vi "Enque Epics Message Bool Array.vi"(7 "Message name":string, 8 "error in (no error)":errorcluster, 9 "Numeric":u32, 10 "Epics variable":bool[](array[boolean]), 11 "Queue in":refnum<queue>) -> (0 "error out":errorcluster)   [LabVIEW 2014]
uses:
  Message Queue/Message Cluster.ctl
  Message Queue/Message Queue.lvlib
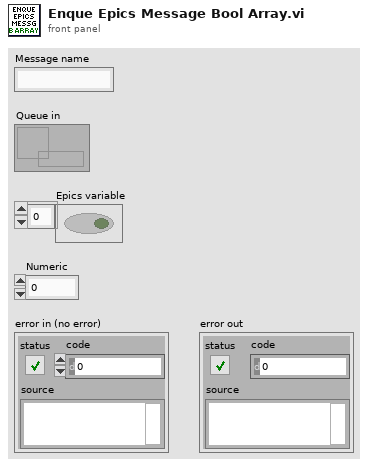
[diagram p1: front panel]
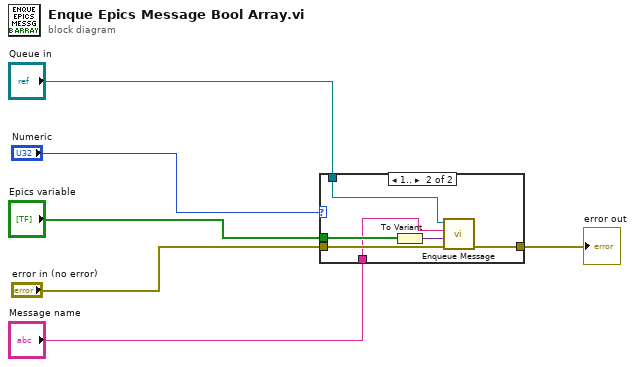
[diagram p0: block diagram]
diagram:
  n1 = case shown="1.." "Numeric" {
    tunnel: "error in (no error)" -> [w7 w13]
    tunnel: [w7 w12] -> w4
    tunnel: "Queue in" -> [_ w11]
    tunnel: "Epics variable" -> [_ w9]
    tunnel: "Message name" -> [_ w8]
    frame 0, Default {
    }
    frame 1.. {
      n2 = To Variant(anything=w9) -> (Variant=w10:variant)
      n3 = call "Enqueue Message.vi"("error in (no error)"=w13, "Message Data"=w10, "Message"=w8, "Message Queue"=w11) -> ("error out"=w12:errorcluster)  [unwired: 6 in, 1 out]
    }
  }
  "error out" <- w4
